vi "Renishaw_XL80_Example.vi"() -> ()   [LabVIEW 2024]
uses:
  Library/Class/Renishaw-XL80/Renishaw-XL80.lvclass
panel:
  out "SerialNo":string
  in  "Get Env Condition":bool
  out "GetHumidity":dbl
  out "pStatus 5":i32(ring) items=["SENSOR_OK"=0, "SENSOR_BAD_READING"=1, "SENSOR_FAILED"=2, "SENSOR_NOT_CONNECTED"=4]
  out "GetPressure":dbl
  out "pStatus 4":i32(ring) items=["SENSOR_OK"=0, "SENSOR_BAD_READING"=1, "SENSOR_FAILED"=2, "SENSOR_NOT_CONNECTED"=4]
  out "GetAirTemp 2":dbl
  out "pStatus 3":i32(ring) items=["SENSOR_OK"=0, "SENSOR_BAD_READING"=1, "SENSOR_FAILED"=2, "SENSOR_NOT_CONNECTED"=4]
  out "Temperature Array":dbl[](array[numeric])
  out "pStatus Array":i32[](array[ring]) items=["SENSOR_OK"=0, "SENSOR_BAD_READING"=1, "SENSOR_FAILED"=2, "SENSOR_NOT_CONNECTED"=4]
  in  "Get MatTemp method":bool
  in  "Air Temp [°C]":dbl
  in  "Humidity [%]":dbl
  in  "Pressure [Pa]":dbl
  in  "Set Update Air Comp2 Method":bool
  out "GetAirTemp":dbl
  out "pStatus 2":i32(ring) items=["SENSOR_OK"=0, "SENSOR_BAD_READING"=1, "SENSOR_FAILED"=2, "SENSOR_NOT_CONNECTED"=4]
  in  "Set ExpansionCoefficient":bool
  in  "ExpansionCoefficient":dbl
  in  "Lambda":dbl
  in  "MatCompFactor":dbl
  in  "Set MatCompFactor":bool
  in  "Set Lambda":bool
  in  "Set AutoCompensationMode":bool
  in  "AutoCompensationMode":i32(ring) items=["AUTO_COMPENSATION_OFF"=0, "AUTO_COMPENSATION_AIR"=1, "AUTO_COMPENSATION_FULL"=3]
  in  "Set MeasurementMode":bool
  in  "MeasurementMode":i32(ring) items=["MEASUREMENT_INDETERMINATE", "MEASUREMENT_LINEAR_PLANE", "MEASUREMENT_LINEAR_RETRO", "MEASUREMENT_ANGULAR", "MEASUREMENT_STRAIGHTNESS_SHORT", "MEASUREMENT_STRAIGHTNESS_LONG", "MEASUREMENT_VELOCITY_RETRO"]
  out "error out 2":errorcluster
  out "error out":errorcluster
  in  "Get Signal Strength":bool
  out "Signal Strength":i16
  in  "Get DX10SerialNumber":bool
  out "DX10SerialNumber":string
  out "OpticsFactor":dbl
  in  "Get OpticsFactor":bool
  in  "Get ML10Version":bool
  out "ML10Version":string
  in  "Get ML10Status":bool
  out "ML10Status":i32(ring)=1 items=["ML10_AVERAGING_ON"=1, "ML10_TPIN_SELECTED"=4, "ML10_BEAM_LOW"=64, "ML10_BEAM_LOSS"=128, "ML10_STABILITY_LOSS"=256, "ML10_PREHEAT"=2048, "ML10_LASER_TOO_COLD"=4096, "ML10_LASER_TOO_HOT"=8192, "ML10_LASER_UNSTABLE"=16384, "ML10_LASER_FAIL"=32768, "ML10_NOT_RESPONDING"=65536, "ML10_LONG_TERM_AVERAGING_ON"=524288, "ML10_MEASUREMENT_MODE"=7340032, "ML10_HIGH_SPEED_ERROR"=8388608, "ML10_DYNAMIC_SELECTED"=16777216]
  out "MeasurementMode":i32(ring) items=["MEASUREMENT_INDETERMINATE", "MEASUREMENT_LINEAR_PLANE", "MEASUREMENT_LINEAR_RETRO", "MEASUREMENT_ANGULAR", "MEASUREMENT_STRAIGHTNESS_SHORT", "MEASUREMENT_STRAIGHTNESS_LONG", "MEASUREMENT_VELOCITY_RETRO"]
  in  "Get MeasurementMode":bool
  in  "Get MatCompFactor":bool
  out "MatCompFactor":dbl
  out "GetLaserMeasurement":dbl format="%_9f"
  out "pStatus":i32(ring) items=["COUNT_OK"=0, "COUNT_ERROR"=1, "COUNT_TPIN_OCCURRED"=2, "COUNT_DATUMED"=4]
  in  "Get Meas data":bool
  in  "Get Lambda":bool
  out "Lambda":dbl
  in  "Get IsConnected":bool
  out "IsConnected":bool
  in  "Get ExpansionCoefficient":bool
  out "ExpansionCoefficient":dbl
  in  "Get EC10Version":bool
  out "EC10Version":string
  out "EC10Status":i32(ring) items=["EC10_CONNECTED"=0, "EC10_NOT_RESPONDING"=65536]
  in  "Get EC10Status":bool
  in  "Get DX10Version":bool
  out "DX10Version":string
  in  "Get DX10Status":bool
  out "DX10Status":i32(ring) items=["DX10_CONNECTED", "DX10_NOT_RESPONDING"]
  out "AutoCompensationMode":i32(ring) items=["AUTO_COMPENSATION_OFF"=0, "AUTO_COMPENSATION_AIR"=1, "AUTO_COMPENSATION_FULL"=3]
  in  "Get AutoCompensationMode":bool
  in  "Get Air Temp":bool
  in  "stop":bool
  out "Serial Number":string
  out "Connect":bool
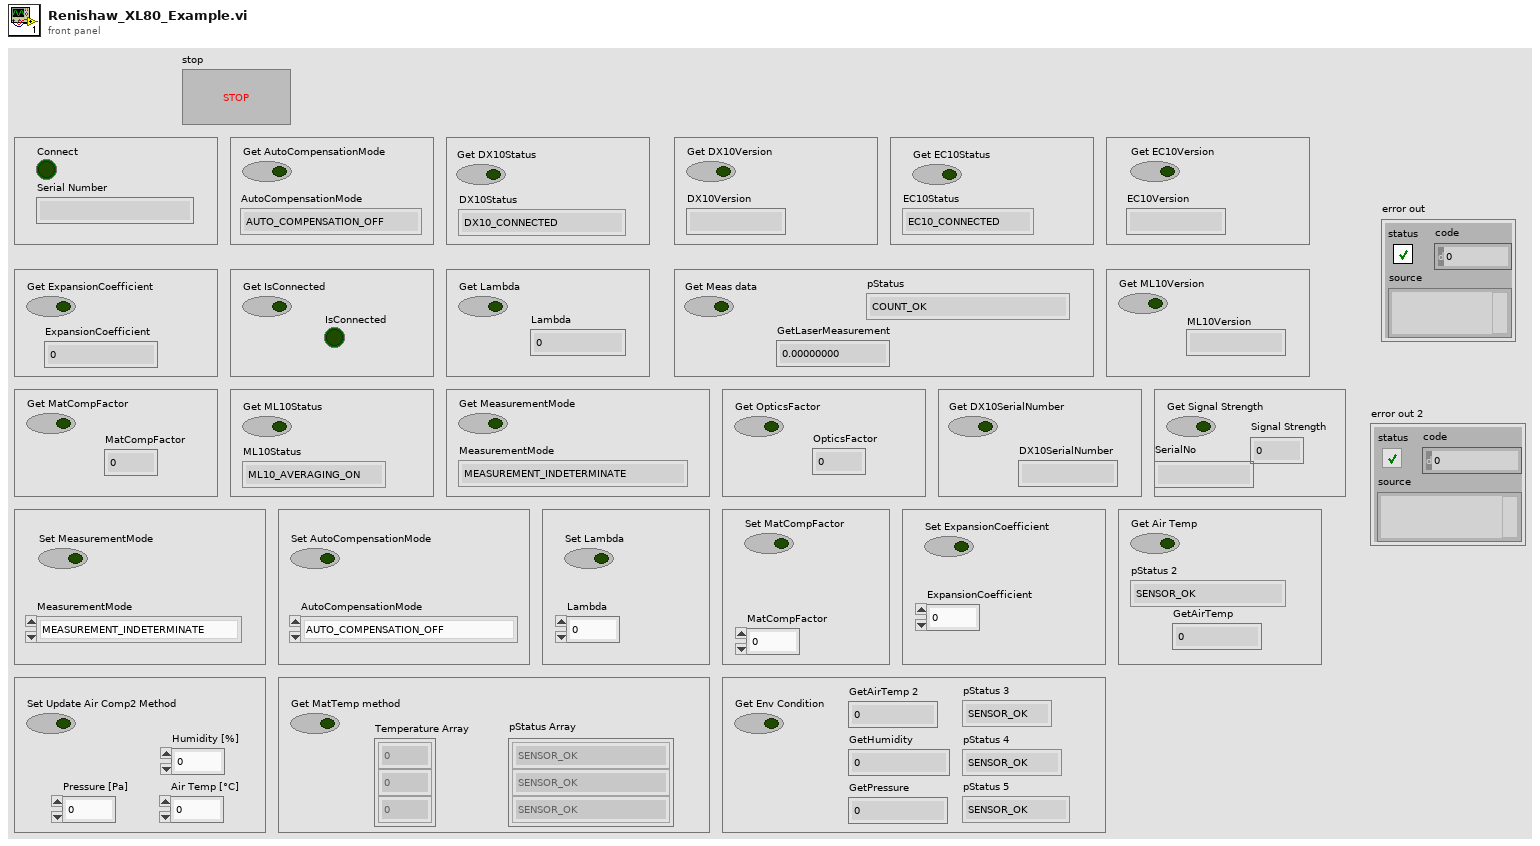
[diagram p1: front panel]
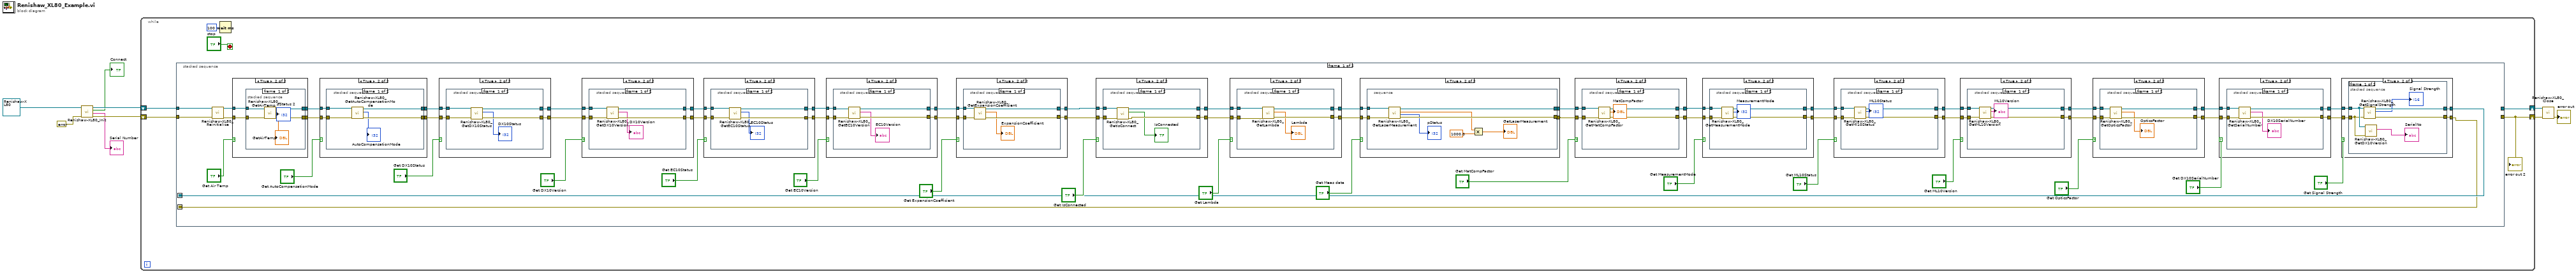
[diagram p0: block diagram]
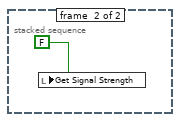
[diagram p3: hidden frame]
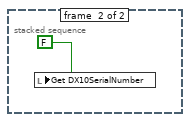
[diagram p5: hidden frame]
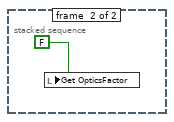
[diagram p7: hidden frame]
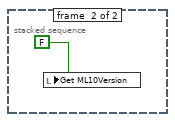
[diagram p9: hidden frame]
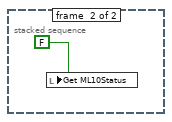
[diagram p11: hidden frame]
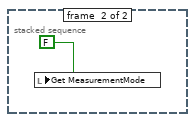
[diagram p13: hidden frame]
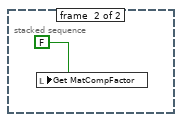
[diagram p15: hidden frame]
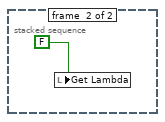
[diagram p18: hidden frame]
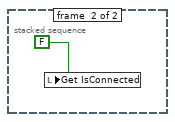
[diagram p20: hidden frame]
diagram:
  n1 = call-dynamic "Renishaw-XL80_Init.vi"("error in (no error)"=errorcluster {"status"=FALSE, "code"=0, "source"=""}, "Renishaw-XL80 in"=refnum<class "Renishaw-XL80.lvclass"> refnum ("Renishaw-XL80.lvclass")) -> ("error out"=w7:errorcluster, "Serial Number"=→"Serial Number":string, "Connect"=→"Connect":bool, "Renishaw-XL80 out"=w8:refnum<class "Renishaw-XL80.lvclass">)  [unwired: 6 in]
  n2 = while {
    shift-right: [w11] -> w4
    shift-left: w8 -> [w13]
    shift-right: [w10] -> w3
    shift-left: w7 -> [w12]
    stop <- "stop" stop-if-true
    n3 = stacked-sequence {
      seq-local: [w17 _] -> [_ w304]
      seq-local: [w16 _] -> [_ w303]
      tunnel: w13 -> [w70 _]
      tunnel: w12 -> [w69 _]
      tunnel: [_ w282] -> w11
      tunnel: [_ w281] -> w10
      frame #0 {
        n4 = call-dynamic "Renishaw-XL80_Reinitialize.vi"("error in (no error)"=w69, "Renishaw-XL80 in"=w70) -> ("error out"=w67:errorcluster, "Renishaw-XL80 out"=w68:refnum<class "Renishaw-XL80.lvclass">)  [unwired: 8 in]
        n5 = case shown="True" "Get Air Temp" {
          tunnel: w68 -> [w267 w271]
          tunnel: w67 -> [w266 w270]
          tunnel: [w267 w269] -> w65
          tunnel: [w266 w268] -> w64
          frame False {
          }
          frame True {
            n6 = stacked-sequence {
              tunnel: w271 -> [w277 _]
              tunnel: w270 -> [w276 _]
              tunnel: [w275 _] -> w269
              tunnel: [w274 _] -> w268
              frame #0 {
                n7 = call-dynamic "Renishaw-XL80_GetAirTemp.vi"("error in (no error)"=w276, "Renishaw-XL80 in"=w277) -> ("error out"=w274:errorcluster, "pStatus"=→"pStatus 2":i32, "GetAirTemp"=→"GetAirTemp":dbl, "Renishaw-XL80 out"=w275:refnum<class "Renishaw-XL80.lvclass">)  [unwired: 6 in]
              }
              frame #1 {
                n8 = local write "Get Air Temp"(FALSE ("Get Air Temp")) -> ()
              }
            }
          }
        }
        n9 = case shown="True" "Get AutoCompensationMode" {
          tunnel: w65 -> [w255 w259]
          tunnel: w64 -> [w254 w258]
          tunnel: [w255 w257] -> w62
          tunnel: [w254 w256] -> w61
          frame False {
          }
          frame True {
            n10 = stacked-sequence {
              tunnel: w259 -> [w264 _]
              tunnel: w258 -> [w261 _]
              tunnel: [w263 _] -> w257
              tunnel: [w262 _] -> w256
              frame #0 {
                n11 = call-dynamic "Renishaw-XL80_GetAutoCompensationMode.vi"("error in (no error)"=w261, "Renishaw-XL80 in"=w264) -> ("error out"=w262:errorcluster, "AutoCompensationMode"=→"AutoCompensationMode":i32, "Renishaw-XL80 out"=w263:refnum<class "Renishaw-XL80.lvclass">)  [unwired: 7 in]
              }
              frame #1 {
                n12 = local write "Get AutoCompensationMode"(FALSE ("Get Air Temp")) -> ()
              }
            }
          }
        }
        n13 = case shown="True" "Get DX10Status" {
          tunnel: w62 -> [w243 w247]
          tunnel: w61 -> [w242 w246]
          tunnel: [w243 w245] -> w59
          tunnel: [w242 w244] -> w58
          frame False {
          }
          frame True {
            n14 = stacked-sequence {
              tunnel: w247 -> [w252 _]
              tunnel: w246 -> [w251 _]
              tunnel: [w249 _] -> w245
              tunnel: [w250 _] -> w244
              frame #0 {
                n15 = call-dynamic "Renishaw-XL80_GetDX10Status.vi"("error in (no error)"=w251, "Renishaw-XL80 in"=w252) -> ("error out"=w250:errorcluster, "DX10Status"=→"DX10Status":i32, "Renishaw-XL80 out"=w249:refnum<class "Renishaw-XL80.lvclass">)  [unwired: 7 in]
              }
              frame #1 {
                n16 = local write "Get DX10Status"(FALSE ("Get Air Temp")) -> ()
              }
            }
          }
        }
        n17 = case shown="True" "Get DX10Version" {
          tunnel: w59 -> [w231 w235]
          tunnel: w58 -> [w230 w234]
          tunnel: [w231 w233] -> w55
          tunnel: [w230 w232] -> w56
          frame False {
          }
          frame True {
            n18 = stacked-sequence {
              tunnel: w235 -> [w240 _]
              tunnel: w234 -> [w239 _]
              tunnel: [w238 _] -> w233
              tunnel: [w237 _] -> w232
              frame #0 {
                n19 = call-dynamic "Renishaw-XL80_GetDX10Version.vi"("error in (no error)"=w239, "Renishaw-XL80 in"=w240) -> ("error out"=w237:errorcluster, "DX10Version"=→"DX10Version":string, "Renishaw-XL80 out"=w238:refnum<class "Renishaw-XL80.lvclass">)  [unwired: 7 in]
              }
              frame #1 {
                n20 = local write "Get DX10Version"(FALSE ("Get Air Temp")) -> ()
              }
            }
          }
        }
        n21 = case shown="True" "Get EC10Status" {
          tunnel: w55 -> [w219 w223]
          tunnel: w56 -> [w218 w222]
          tunnel: [w219 w220] -> w52
          tunnel: [w218 w221] -> w53
          frame False {
          }
          frame True {
            n22 = stacked-sequence {
              tunnel: w223 -> [w228 _]
              tunnel: w222 -> [w227 _]
              tunnel: [w226 _] -> w221
              tunnel: [w225 _] -> w220
              frame #0 {
                n23 = call-dynamic "Renishaw-XL80_GetEC10Status.vi"("error in (no error)"=w227, "Renishaw-XL80 in"=w228) -> ("error out"=w226:errorcluster, "EC10Status"=→"EC10Status":i32, "Renishaw-XL80 out"=w225:refnum<class "Renishaw-XL80.lvclass">)  [unwired: 7 in]
              }
              frame #1 {
                n24 = local write "Get EC10Status"(FALSE ("Get Air Temp")) -> ()
              }
            }
          }
        }
        n25 = case shown="True" "Get EC10Version" {
          tunnel: w52 -> [w207 w211]
          tunnel: w53 -> [w206 w210]
          tunnel: [w207 w209] -> w50
          tunnel: [w206 w208] -> w49
          frame False {
          }
          frame True {
            n26 = stacked-sequence {
              tunnel: w211 -> [w215 _]
              tunnel: w210 -> [w216 _]
              tunnel: [w214 _] -> w209
              tunnel: [w213 _] -> w208
              frame #0 {
                n27 = call-dynamic "Renishaw-XL80_GetEC10Version.vi"("error in (no error)"=w216, "Renishaw-XL80 in"=w215) -> ("error out"=w213:errorcluster, "EC10Version"=→"EC10Version":string, "Renishaw-XL80 out"=w214:refnum<class "Renishaw-XL80.lvclass">)  [unwired: 7 in]
              }
              frame #1 {
                n28 = local write "Get EC10Status"(FALSE ("Get Air Temp")) -> ()
              }
            }
          }
        }
        n29 = case shown="True" "Get ExpansionCoefficient" {
          tunnel: w50 -> [w195 w199]
          tunnel: w49 -> [w194 w198]
          tunnel: [w195 w197] -> w46
          tunnel: [w194 w196] -> w47
          frame False {
          }
          frame True {
            n30 = stacked-sequence {
              tunnel: w199 -> [w204 _]
              tunnel: w198 -> [w203 _]
              tunnel: [w201 _] -> w197
              tunnel: [w202 _] -> w196
              frame #0 {
                n31 = call-dynamic "Renishaw-XL80_GetExpansionCoefficient.vi"("error in (no error)"=w203, "Renishaw-XL80 in"=w204) -> ("error out"=w202:errorcluster, "ExpansionCoefficient"=→"ExpansionCoefficient":dbl, "Renishaw-XL80 out"=w201:refnum<class "Renishaw-XL80.lvclass">)  [unwired: 7 in]
              }
              frame #1 {
                n32 = local write "Get ExpansionCoefficient"(FALSE ("Get Air Temp")) -> ()
              }
            }
          }
        }
        n33 = case shown="True" "Get IsConnected" {
          tunnel: w46 -> [w183 w187]
          tunnel: w47 -> [w182 w186]
          tunnel: [w183 w185] -> w44
          tunnel: [w182 w184] -> w43
          frame False {
          }
          frame True {
            n34 = stacked-sequence {
              tunnel: w187 -> [w192 _]
              tunnel: w186 -> [w191 _]
              tunnel: [w189 _] -> w185
              tunnel: [w190 _] -> w184
              frame #0 {
                n35 = call-dynamic "Renishaw-XL80_GetIsConnect.vi"("error in (no error)"=w191, "Renishaw-XL80 in"=w192) -> ("error out"=w190:errorcluster, "IsConnected"=→"IsConnected":bool, "Renishaw-XL80 out"=w189:refnum<class "Renishaw-XL80.lvclass">)  [unwired: 7 in]
              }
              frame #1 {
                n36 = local write "Get IsConnected"(FALSE ("Get Air Temp")) -> ()
              }
            }
          }
        }
        n37 = case shown="True" "Get Lambda" {
          tunnel: w44 -> [w171 w175]
          tunnel: w43 -> [w170 w174]
          tunnel: [w171 w173] -> w41
          tunnel: [w170 w172] -> w40
          frame False {
          }
          frame True {
            n38 = stacked-sequence {
              tunnel: w175 -> [w180 _]
              tunnel: w174 -> [w179 _]
              tunnel: [w178 _] -> w173
              tunnel: [w177 _] -> w172
              frame #0 {
                n39 = call-dynamic "Renishaw-XL80_GetLambda.vi"("error in (no error)"=w179, "Renishaw-XL80 in"=w180) -> ("error out"=w177:errorcluster, "Lambda"=→"Lambda":dbl, "Renishaw-XL80 out"=w178:refnum<class "Renishaw-XL80.lvclass">)  [unwired: 7 in]
              }
              frame #1 {
                n40 = local write "Get Lambda"(FALSE ("Get Air Temp")) -> ()
              }
            }
          }
        }
        n41 = case shown="True" "Get Meas data" {
          tunnel: w41 -> [w157 w161]
          tunnel: w40 -> [w156 w160]
          tunnel: [w157 w159] -> w38
          tunnel: [w156 w158] -> w37
          frame False {
          }
          frame True {
            n42 = stacked-sequence {
              tunnel: w161 -> [w169]
              tunnel: w160 -> [w168]
              tunnel: [w167] -> w159
              tunnel: [w166] -> w158
              frame #0 {
                n43 = call-dynamic "Renishaw-XL80_GetLaserMeasurement.vi"("error in (no error)"=w168, "Renishaw-XL80 in"=w169) -> ("error out"=w166:errorcluster, "pStatus"=→"pStatus":i32, "GetLaserMeasurement"=w164:dbl, "Renishaw-XL80 out"=w167:refnum<class "Renishaw-XL80.lvclass">)  [unwired: 6 in]
                n44 = Multiply(x=w164, y=1000.0) -> (x*y=→"GetLaserMeasurement":dbl)
              }
            }
          }
        }
        n45 = case shown="True" "Get MatCompFactor" {
          tunnel: w38 -> [w145 w149]
          tunnel: w37 -> [w144 w148]
          tunnel: [w145 w147] -> w35
          tunnel: [w144 w146] -> w34
          frame False {
          }
          frame True {
            n46 = stacked-sequence {
              tunnel: w149 -> [w154 _]
              tunnel: w148 -> [w153 _]
              tunnel: [w152 _] -> w147
              tunnel: [w151 _] -> w146
              frame #0 {
                n47 = call-dynamic "Renishaw-XL80_GetMatCompFactor.vi"("error in (no error)"=w153, "Renishaw-XL80 in"=w154) -> ("error out"=w151:errorcluster, "MatCompFactor"=→"MatCompFactor":dbl, "Renishaw-XL80 out"=w152:refnum<class "Renishaw-XL80.lvclass">)  [unwired: 7 in]
              }
              frame #1 {
                n48 = local write "Get MatCompFactor"(FALSE ("Get Air Temp")) -> ()
              }
            }
          }
        }
        n49 = case shown="True" "Get MeasurementMode" {
          tunnel: w35 -> [w133 w137]
          tunnel: w34 -> [w132 w136]
          tunnel: [w133 w135] -> w32
          tunnel: [w132 w134] -> w31
          frame False {
          }
          frame True {
            n50 = stacked-sequence {
              tunnel: w137 -> [w142 _]
              tunnel: w136 -> [w141 _]
              tunnel: [w140 _] -> w135
              tunnel: [w139 _] -> w134
              frame #0 {
                n51 = call-dynamic "Renishaw-XL80_GetMeasurementMode.vi"("error in (no error)"=w141, "Renishaw-XL80 in"=w142) -> ("error out"=w139:errorcluster, "MeasurementMode"=→"MeasurementMode":i32, "Renishaw-XL80 out"=w140:refnum<class "Renishaw-XL80.lvclass">)  [unwired: 7 in]
              }
              frame #1 {
                n52 = local write "Get MeasurementMode"(FALSE ("Get Air Temp")) -> ()
              }
            }
          }
        }
        n53 = case shown="True" "Get ML10Status" {
          tunnel: w32 -> [w121 w125]
          tunnel: w31 -> [w120 w124]
          tunnel: [w121 w123] -> w29
          tunnel: [w120 w122] -> w28
          frame False {
          }
          frame True {
            n54 = stacked-sequence {
              tunnel: w125 -> [w130 _]
              tunnel: w124 -> [w129 _]
              tunnel: [w127 _] -> w123
              tunnel: [w128 _] -> w122
              frame #0 {
                n55 = call-dynamic "Renishaw-XL80_GetMl10Status.vi"("error in (no error)"=w129, "Renishaw-XL80 in"=w130) -> ("error out"=w128:errorcluster, "ML10Status"=→"ML10Status":i32, "Renishaw-XL80 out"=w127:refnum<class "Renishaw-XL80.lvclass">)  [unwired: 7 in]
              }
              frame #1 {
                n56 = local write "Get ML10Status"(FALSE ("Get Air Temp")) -> ()
              }
            }
          }
        }
        n57 = case shown="True" "Get ML10Version" {
          tunnel: w29 -> [w109 w113]
          tunnel: w28 -> [w108 w112]
          tunnel: [w109 w111] -> w26
          tunnel: [w108 w110] -> w25
          frame False {
          }
          frame True {
            n58 = stacked-sequence {
              tunnel: w113 -> [w118 _]
              tunnel: w112 -> [w117 _]
              tunnel: [w116 _] -> w111
              tunnel: [w115 _] -> w110
              frame #0 {
                n59 = call-dynamic "Renishaw-XL80_GetML10Version.vi"("error in (no error)"=w117, "Renishaw-XL80 in"=w118) -> ("error out"=w115:errorcluster, "ML10Version"=→"ML10Version":string, "Renishaw-XL80 out"=w116:refnum<class "Renishaw-XL80.lvclass">)  [unwired: 7 in]
              }
              frame #1 {
                n60 = local write "Get ML10Version"(FALSE ("Get Air Temp")) -> ()
              }
            }
          }
        }
        n61 = case shown="True" "Get OpticsFactor" {
          tunnel: w26 -> [w97 w101]
          tunnel: w25 -> [w96 w100]
          tunnel: [w97 w99] -> w22
          tunnel: [w96 w98] -> w23
          frame False {
          }
          frame True {
            n62 = stacked-sequence {
              tunnel: w101 -> [w105 _]
              tunnel: w100 -> [w106 _]
              tunnel: [w103 _] -> w99
              tunnel: [w104 _] -> w98
              frame #0 {
                n63 = call-dynamic "Renishaw-XL80_GetOpticsFactor.vi"("error in (no error)"=w106, "Renishaw-XL80 in"=w105) -> ("error out"=w104:errorcluster, "OpticsFactor"=→"OpticsFactor":dbl, "Renishaw-XL80 out"=w103:refnum<class "Renishaw-XL80.lvclass">)  [unwired: 7 in]
              }
              frame #1 {
                n64 = local write "Get OpticsFactor"(FALSE ("Get Air Temp")) -> ()
              }
            }
          }
        }
        n65 = case shown="True" "Get DX10SerialNumber" {
          tunnel: w22 -> [w85 w89]
          tunnel: w23 -> [w84 w88]
          tunnel: [w85 w87] -> w19
          tunnel: [w84 w86] -> w20
          frame False {
          }
          frame True {
            n66 = stacked-sequence {
              tunnel: w89 -> [w94 _]
              tunnel: w88 -> [w93 _]
              tunnel: [w92 _] -> w87
              tunnel: [w91 _] -> w86
              frame #0 {
                n67 = call-dynamic "Renishaw-XL80_GetSerialNumber.vi"("error in (no error)"=w93, "Renishaw-XL80 in"=w94) -> ("error out"=w91:errorcluster, "DX10SerialNumber"=→"DX10SerialNumber":string, "Renishaw-XL80 out"=w92:refnum<class "Renishaw-XL80.lvclass">)  [unwired: 7 in]
              }
              frame #1 {
                n68 = local write "Get DX10SerialNumber"(FALSE ("Get Air Temp")) -> ()
              }
            }
          }
        }
        n69 = case shown="True" "Get Signal Strength" {
          tunnel: w19 -> [w72 w76]
          tunnel: w20 -> [w71 w75]
          tunnel: [w72 w74] -> w17
          tunnel: [w71 w73] -> w16
          frame False {
          }
          frame True {
            n70 = stacked-sequence {
              tunnel: w76 -> [w79 _]
              tunnel: w75 -> [w78 _]
              tunnel: [w81 _] -> w74
              tunnel: [w82 _] -> w73
              frame #0 {
                n71 = call-dynamic "Renishaw-XL80_GetSignalStrength.vi"("error in (no error)"=w78, "Renishaw-XL80 in"=w79) -> ("error out"=w82:errorcluster, "Signal Strength"=→"Signal Strength":i16, "Renishaw-XL80 out"=w81:refnum<class "Renishaw-XL80.lvclass">)  [unwired: 7 in]
                n72 = call-dynamic "Renishaw-XL80_GetDX10Version.vi"("error in (no error)"=w78, "Renishaw-XL80 in"=w79) -> ("DX10Version"=→"SerialNo":string)  [unwired: 7 in, 2 out]
              }
              frame #1 {
                n73 = local write "Get Signal Strength"(FALSE ("Get Air Temp")) -> ()
              }
            }
          }
        }
      }
      frame #1 {
        n74 = case shown="True" "Set MeasurementMode" {
          tunnel: w304 -> [w402 w406]
          tunnel: w303 -> [w401 w405]
          tunnel: [w402 w404] -> w301
          tunnel: [w401 w403] -> w300
          frame False {
          }
          frame True {
            n75 = stacked-sequence {
              tunnel: w406 -> [w409 _]
              tunnel: w405 -> [w408 _]
              tunnel: [w411 _] -> w404
              tunnel: [w410 _] -> w403
              frame #0 {
                n76 = call-dynamic "Renishaw-XL80_SetMeasurementMode.vi"("error in (no error)"=w408, "MeasurementMode"="MeasurementMode", "Renishaw-XL80 in"=w409) -> ("error out"=w410:errorcluster, "Renishaw-XL80 out"=w411:refnum<class "Renishaw-XL80.lvclass">)  [unwired: 7 in]
              }
              frame #1 {
                n77 = local write "Set MeasurementMode"(FALSE ("Get Air Temp")) -> ()
              }
            }
          }
        }
        n78 = case shown="True" "Set AutoCompensationMode" {
          tunnel: w301 -> [w390 w394]
          tunnel: w300 -> [w389 w393]
          tunnel: [w390 w392] -> w298
          tunnel: [w389 w391] -> w297
          frame False {
          }
          frame True {
            n79 = stacked-sequence {
              tunnel: w394 -> [w399 _]
              tunnel: w393 -> [w398 _]
              tunnel: [w396 _] -> w392
              tunnel: [w397 _] -> w391
              frame #0 {
                n80 = call-dynamic "Renishaw-XL80_SetAutoCompensationMode.vi"("error in (no error)"=w398, "AutoCompensationMode"="AutoCompensationMode", "Renishaw-XL80 in"=w399) -> ("error out"=w397:errorcluster, "Renishaw-XL80 out"=w396:refnum<class "Renishaw-XL80.lvclass">)  [unwired: 7 in]
              }
              frame #1 {
                n81 = local write "Set AutoCompensationMode"(FALSE ("Get Air Temp")) -> ()
              }
            }
          }
        }
        n82 = case shown="True" "Set Lambda" {
          tunnel: w298 -> [w378 w382]
          tunnel: w297 -> [w377 w381]
          tunnel: [w378 w380] -> w295
          tunnel: [w377 w379] -> w294
          frame False {
          }
          frame True {
            n83 = stacked-sequence {
              tunnel: w382 -> [w385 _]
              tunnel: w381 -> [w384 _]
              tunnel: [w387 _] -> w380
              tunnel: [w386 _] -> w379
              frame #0 {
                n84 = call-dynamic "Renishaw-XL80_SetLambda.vi"("error in (no error)"=w384, "Lambda"="Lambda", "Renishaw-XL80 in"=w385) -> ("error out"=w386:errorcluster, "Renishaw-XL80 out"=w387:refnum<class "Renishaw-XL80.lvclass">)  [unwired: 7 in]
              }
              frame #1 {
                n85 = local write "Set Lambda"(FALSE ("Get Air Temp")) -> ()
              }
            }
          }
        }
        n86 = case shown="True" "Set MatCompFactor" {
          tunnel: w295 -> [w366 w370]
          tunnel: w294 -> [w365 w369]
          tunnel: [w366 w368] -> w292
          tunnel: [w365 w367] -> w291
          frame False {
          }
          frame True {
            n87 = stacked-sequence {
              tunnel: w370 -> [w373 _]
              tunnel: w369 -> [w372 _]
              tunnel: [w374 _] -> w368
              tunnel: [w375 _] -> w367
              frame #0 {
                n88 = call-dynamic "Renishaw-XL80_SetMatCompFactor.vi"("error in (no error)"=w372, "MatCompFactor"="MatCompFactor", "Renishaw-XL80 in"=w373) -> ("error out"=w375:errorcluster, "Renishaw-XL80 out"=w374:refnum<class "Renishaw-XL80.lvclass">)  [unwired: 7 in]
              }
              frame #1 {
                n89 = local write "Set MatCompFactor"(FALSE ("Get Air Temp")) -> ()
              }
            }
          }
        }
        n90 = case shown="True" "Set ExpansionCoefficient" {
          tunnel: w292 -> [w354 w358]
          tunnel: w291 -> [w353 w357]
          tunnel: [w354 w356] -> w289
          tunnel: [w353 w355] -> w288
          frame False {
          }
          frame True {
            n91 = stacked-sequence {
              tunnel: w358 -> [w360 _]
              tunnel: w357 -> [w361 _]
              tunnel: [w362 _] -> w356
              tunnel: [w363 _] -> w355
              frame #0 {
                n92 = call-dynamic "Renishaw-XL80_SetExpansionCoefficient.vi"("error in (no error)"=w361, "ExpansionCoefficient"="ExpansionCoefficient", "Renishaw-XL80 in"=w360) -> ("error out"=w363:errorcluster, "Renishaw-XL80 out"=w362:refnum<class "Renishaw-XL80.lvclass">)  [unwired: 7 in]
              }
              frame #1 {
                n93 = local write "Set ExpansionCoefficient"(FALSE ("Get Air Temp")) -> ()
              }
            }
          }
        }
        n94 = case shown="True" "Set Update Air Comp2 Method" {
          tunnel: w289 -> [w340 w344]
          tunnel: [w340 w343] -> w286
          tunnel: [w339 w342] -> w285
          tunnel: w288 -> [w339 w341]
          frame False {
          }
          frame True {
            n95 = stacked-sequence {
              tunnel: w344 -> [w351 _]
              tunnel: [w350 _] -> w343
              tunnel: [w349 _] -> w342
              tunnel: w341 -> [w348 _]
              frame #0 {
                n96 = call-dynamic "Renishaw-XL80_SetUpdateAirCompMethod2.vi"("Pressure [Pa]"="Pressure [Pa]", "error in (no error)"=w348, "Humidity [%]"="Humidity [%]", "Air Temp [°C]"="Air Temp [°C]", "Renishaw-XL80 in"=w351) -> ("error out"=w349:errorcluster, "Renishaw-XL80 out"=w350:refnum<class "Renishaw-XL80.lvclass">)  [unwired: 5 in]
              }
              frame #1 {
                n97 = local write "Set Update Air Comp2 Method"(FALSE ("Set Update Air Comp2 Method")) -> ()
              }
            }
          }
        }
        n98 = case shown="True" "Get MatTemp method" {
          tunnel: w286 -> [w327 w331]
          tunnel: [w327 w330] -> w283
          tunnel: [w326 w329] -> w280
          tunnel: w285 -> [w326 w328]
          frame False {
          }
          frame True {
            n99 = stacked-sequence {
              tunnel: w331 -> [w337 _]
              tunnel: [w336 _] -> w330
              tunnel: [w334 _] -> w329
              tunnel: w328 -> [w335 _]
              frame #0 {
                n100 = call-dynamic "Renishaw-XL80_GetMatTemp.vi"("error in (no error)"=w335, "Renishaw-XL80 in"=w337) -> ("error out"=w334:errorcluster, "pStatus Array"=→"pStatus Array":i32[], "Temperature Array"=→"Temperature Array":dbl[], "Renishaw-XL80 out"=w336:refnum<class "Renishaw-XL80.lvclass">)  [unwired: 6 in]
              }
              frame #1 {
                n101 = local write "Get MatTemp method"(FALSE ("Get MatTemp method")) -> ()
              }
            }
          }
        }
        n102 = case shown="True" "Get Env Condition" {
          tunnel: w283 -> [w306 w310]
          tunnel: [w306 w309] -> w282
          tunnel: [w305 w308] -> w281
          tunnel: w280 -> [w305 w307]
          frame False {
          }
          frame True {
            n103 = stacked-sequence {
              tunnel: w310 -> [w324 _]
              tunnel: [w322 _] -> w309
              tunnel: [w321 _] -> w308
              tunnel: w307 -> [w323 _]
              frame #0 {
                n104 = call-dynamic "Renishaw-XL80_GetHumidity.vi"("error in (no error)"=w323, "Renishaw-XL80 in"=w324) -> ("error out"=w319:errorcluster, "pStatus"=→"pStatus 5":i32, "GetHumidity"=→"GetHumidity":dbl, "Renishaw-XL80 out"=w320:refnum<class "Renishaw-XL80.lvclass">)  [unwired: 6 in]
                n105 = call-dynamic "Renishaw-XL80_GetAirTemp.vi"("error in (no error)"=w319, "Renishaw-XL80 in"=w320) -> ("error out"=w317:errorcluster, "pStatus"=→"pStatus 3":i32, "GetAirTemp"=→"GetAirTemp 2":dbl, "Renishaw-XL80 out"=w318:refnum<class "Renishaw-XL80.lvclass">)  [unwired: 6 in]
                n106 = call-dynamic "Renishaw-XL80_GetPressure.vi"("error in (no error)"=w317, "Renishaw-XL80 in"=w318) -> ("error out"=w321:errorcluster, "pStatus"=→"pStatus 4":i32, "GetPressure"=→"GetPressure":dbl, "Renishaw-XL80 out"=w322:refnum<class "Renishaw-XL80.lvclass">)  [unwired: 6 in]
              }
              frame #1 {
                n107 = local write "Get Env Condition"(FALSE ("Get Env Condition")) -> ()
              }
            }
          }
        }
      }
    }
    "error out 2" <- w10
    n108 = Wait (ms)(milliseconds to wait=u32 100) -> ()  [unwired: 1 out]
  }
  n109 = call-dynamic "Renishaw-XL80_Close.vi"("error in (no error)"=w3, "Renishaw-XL80 in"=w4) -> ("error out"=→"error out":errorcluster)  [unwired: 8 in, 1 out]
